vi "Read Addr.vi"(8 "error in (no error)":errorcluster, 11 "Lakeshore 336 in":refnum<class "Lakeshore 336.lvclass">) -> (0 "error out":errorcluster, 2 "Addr":refnum<visa-resource-name>, 3 "Lakeshore 336 out":refnum<class "Lakeshore 336.lvclass">)   [LabVIEW 2022 SP3, in "Lakeshore 336.lvclass"]
uses:
  Lakeshore 336.lvclass
  Lakeshore 336.lvclass/Lakeshore 336.ctl
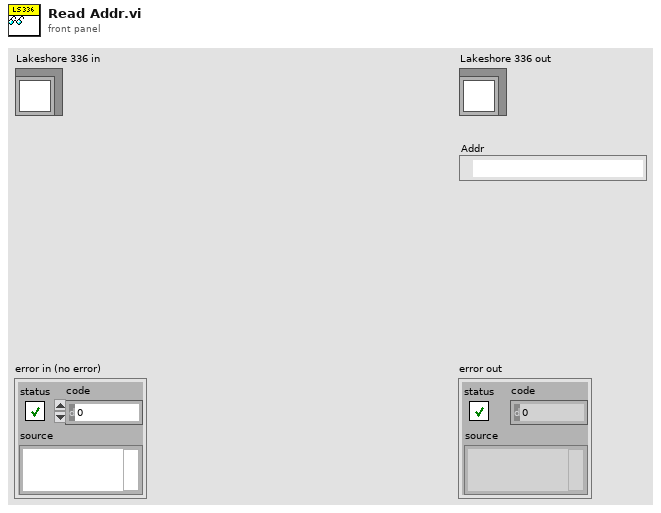
[diagram p1: front panel]
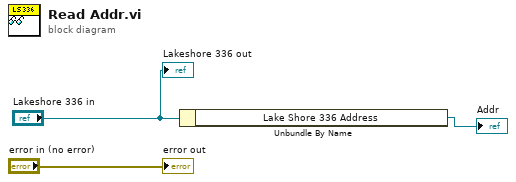
[diagram p0: block diagram]
diagram:
  n1 = Unbundle By Name("Lakeshore 336 in") -> ("Lake Shore 336 Address"=→"Addr":refnum<visa-resource-name>)
  "error out" <- "error in (no error)"
  "Lakeshore 336 out" <- "Lakeshore 336 in"
